vi "Acquire Null Offset For Limit Test.vi"(8 "error in (no error)":errorcluster, 10 "Channel (0: Channel 1)":i32(ring) items=["Channel 1", "Channel 2"], 11 "VISA resource name":refnum<visa-resource-name>) -> (0 "error out":errorcluster, 2 "Acquired Null Offset":dbl, 3 "VISA resource name out":refnum<visa-resource-name>)   [LabVIEW 2020, in "Agilent B2900 Series.lvlib"]
doc: "Automatically set the null offset value used for calculating the limit test data.\nThe null offset value will be the present available value of the latest limit test data. Or it is 0.0 if the present available value does not exist.\n\n<B>Note:</B> \n(1) Use this VI only with other low-level VIs. The high-level VIs automatically incorporate this functionality. This VI does not check the instrument status. \n(2) This VI is not applicable for Agilent models B2961A, B2962A, B2961B, B2962B, B2961C and B2962C."
uses:
  Agilent B2900 Series.lvlib
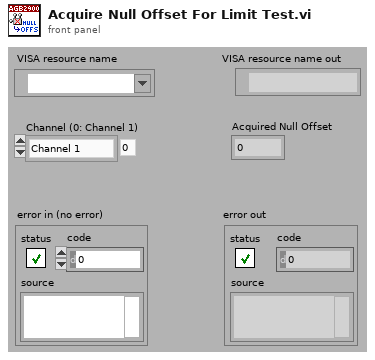
[diagram p1: front panel]
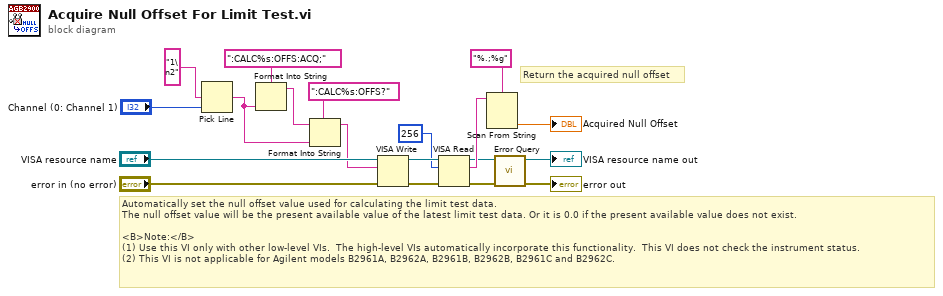
[diagram p0: block diagram]
diagram:
  # "Automatically set the null offset value used for calculating the limit test data.\nThe null offset value will be the present available value of the latest limit test data. Or it is 0.0 if the present available value does not exist.\n\n<B>Note:</B> \n(1) Use this VI only with other low-level VIs.  The high-level VIs automatically incorporate this functionality.  This VI does not check the instrument status.   \n(2) This VI is not applicable for Agilent models B2961A, B2962A, B2961B, B2962B, B2961C and B2962C."
  # "Return the acquired null offset"
  n1 = Pick Line(multi-line string="1\n2" ("string (\"\")"), line index="Channel (0: Channel 1)") -> (output string=w12:string)  [unwired: 1 in]
  n2 = Format Into String(format string=":CALC%s:OFFS:ACQ;", w12) -> (resulting string=w14:string)  [unwired: 2 in, 1 out]
  n3 = Format Into String(format string=":CALC%s:OFFS?", initial string=w14, w12) -> (resulting string=w11:string)  [unwired: 1 in, 1 out]
  n4 = VISA Write(VISA resource name="VISA resource name", write buffer=w11, error in (no error)="error in (no error)") -> (VISA resource name out=w9:refnum<visa-resource-name>, error out=w10:errorcluster)  [unwired: 1 out]
  n5 = VISA Read(VISA resource name=w9, byte count=u32 256, error in (no error)=w10) -> (VISA resource name out=w4:refnum<visa-resource-name>, read buffer=w7:string, error out=w3:errorcluster)  [unwired: 1 out]
  n6 = Scan From String(format string="%.;%g", input string=w7) -> (output 1=→"Acquired Null Offset":dbl)  [unwired: 3 in, 3 out]
  n7 = call "Error Query.vi"("error in (no error)"=w3, "VISA resource name"=w4) -> ("error out"=→"error out":errorcluster, "VISA resource name out"=→"VISA resource name out":refnum<visa-resource-name>)  [unwired: 6 in, 2 out]
